vi "Write Requests.vi"(8 "error in (no error)":errorcluster, 10 "Requests":string[](array[string]), 11 "Personnel in":refnum<class "Personnel.lvclass">) -> (0 "error out":errorcluster, 3 "Personnel out":refnum<class "Personnel.lvclass">)   [LabVIEW 2015, in "Personnel.lvclass"]
uses:
  Personnel.lvclass
  Personnel.lvclass/Personnel.ctl
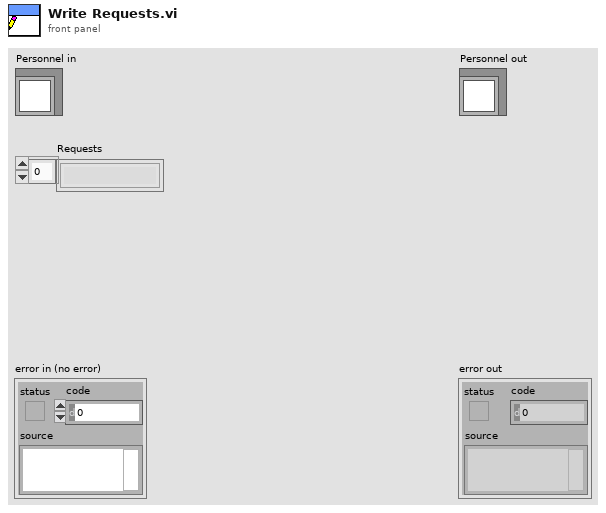
[diagram p1: front panel]
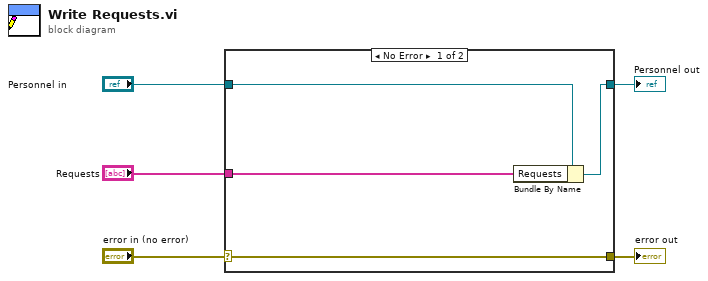
[diagram p0: block diagram]
diagram:
  n1 = case shown="No Error" "error in (no error)" {
    selector: "error in (no error)" -> [w9 w10]
    tunnel: [w9 w10] -> w4
    tunnel: [w7 w11] -> w2
    tunnel: "Personnel in" -> [w8 w11]
    tunnel: "Requests" -> [w6 _]
    frame No Error {
      n2 = Bundle By Name(cluster=w8, "Requests"=w6) -> (w7:refnum<class "Personnel.lvclass">)
    }
    frame Error {
    }
  }
  "error out" <- w4
  "Personnel out" <- w2
